vi "TCP Factory.vi"(8 "error in (no error)":errorcluster, 10 "TCP settings":T1) -> (0 "error out":errorcluster, 3 "protocol out":refnum<class "Protocol Parent.lvclass">)   [LabVIEW 2023, in "Protocols.lvlib" / "TCP.lvclass"]
doc: "Instantiates a new TCP Protocol object using the provided TCP settings."
uses:
  TCP.lvclass
  Protocol Parent/Protocol Parent.lvclass
  TCP Settings.ctl
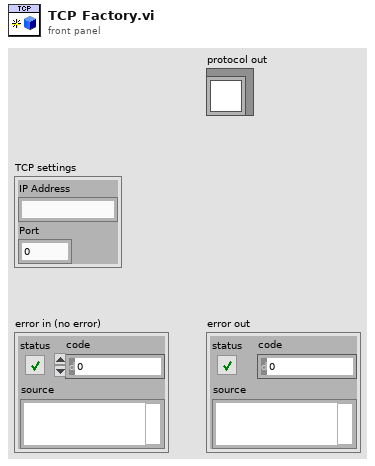
[diagram p1: front panel]
types:
  T1 = typedef "Protocols.lvlib/TCP.lvclass/TCP Settings.ctl" = cluster{"IP Address":string, "Port":u16}
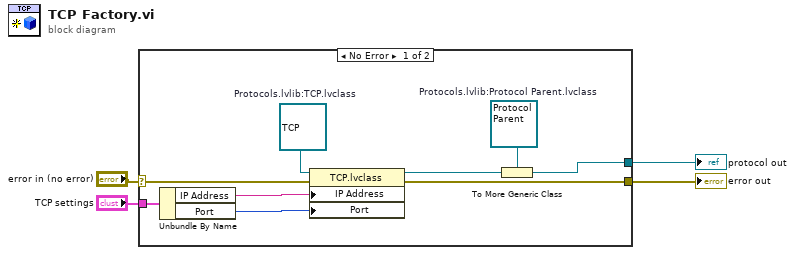
[diagram p0: block diagram]
diagram:
  n1 = case shown="No Error" "error in (no error)" {
    selector: "error in (no error)" -> [w8 w14]
    tunnel: "TCP settings" -> [w13 _]
    tunnel: [w9 w14] -> w3
    tunnel: [w6 _] -> w1
    frame No Error {
      w5 = refnum<class "Protocol Parent.lvclass"> refnum  # Protocols.lvlib:Protocol Parent.lvclass
      w12 = refnum<class "TCP.lvclass"> refnum  # Protocols.lvlib:TCP.lvclass
      n2 = Unbundle By Name(w13) -> ("IP Address"=w11:string, "Port"=w10:u16)
      n3 = property class="TCP.lvclass"(reference=w12, error in=w8, "IP Address"=w11, "Port"=w10) -> (reference out=w7:refnum<class "TCP.lvclass">, error out=w9:errorcluster)
      n4 = To More Generic Class(target class=w5, reference=w7) -> (generic class reference=w6:refnum<class "Protocol Parent.lvclass">)
    }
    frame Error {
    }
  }
  "error out" <- w3
  "protocol out" <- w1
